vi "Inficon_Manual_HHV.vi"(5 "HHV-NG-Manual":sgl=1069.0, 6 "Manual HHV":bool, 7 "HHV-LP-Manual":sgl=2548.0, 8 "error in (no error)":errorcluster, 10 "Inficon_LP":refnum<queue>, 11 "Inficon_NG":refnum<queue>) -> (0 "error out":errorcluster)   [LabVIEW 2023]
uses:
  Tenney/support/Message Queue/Message Cluster.ctl
  Tenney/support/Message Queue/Enqueue Message (Single).vi
  Tenney/support/Message Queue/Tenney Message Queue.lvlib
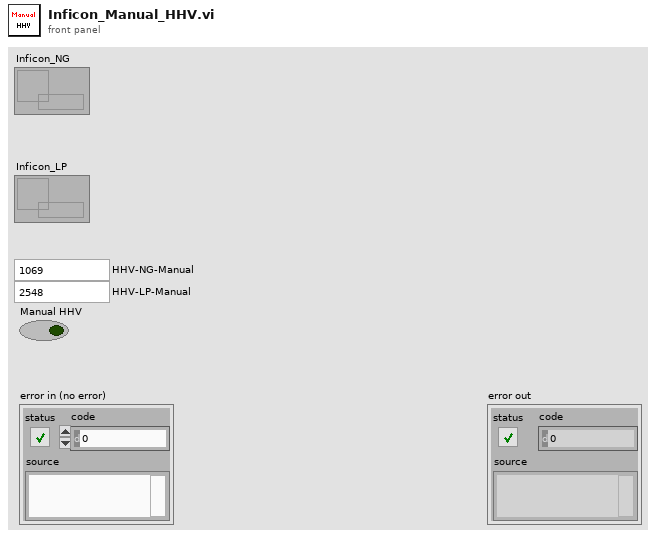
[diagram p1: front panel]
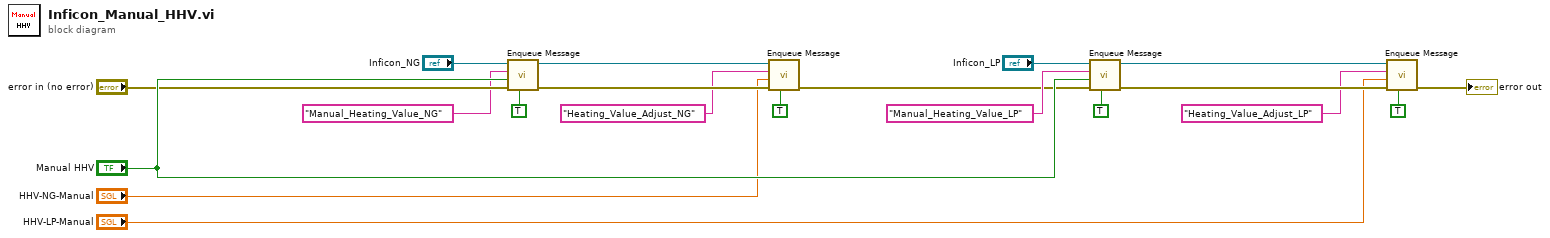
[diagram p0: block diagram]
diagram:
  n1 = call-poly "Enqueue Message.vi"("Priority Message? (F)"=TRUE, "error in (no error)"="error in (no error)", "Message Data"="Manual HHV", "Message"="Manual_Heating_Value_NG", "Message Queue"="Inficon_NG") -> ("error out"=w11:errorcluster, "dup Message Queue"=w9:refnum<queue>)  [unwired: 5 in]
  n2 = call-poly "Enqueue Message.vi"("Priority Message? (F)"=TRUE, "error in (no error)"=w11, "Message Data"="HHV-NG-Manual", "Message"="Heating_Value_Adjust_NG", "Message Queue"=w9) -> ("error out"=w10:errorcluster)  [unwired: 5 in, 1 out]
  n3 = call-poly "Enqueue Message.vi"("Priority Message? (F)"=TRUE, "error in (no error)"=w10, "Message Data"="Manual HHV", "Message"="Manual_Heating_Value_LP", "Message Queue"="Inficon_LP") -> ("error out"=w6:errorcluster, "dup Message Queue"=w5:refnum<queue>)  [unwired: 5 in]
  n4 = call-poly "Enqueue Message.vi"("Priority Message? (F)"=TRUE, "error in (no error)"=w6, "Message Data"="HHV-LP-Manual", "Message"="Heating_Value_Adjust_LP", "Message Queue"=w5) -> ("error out"=→"error out":errorcluster)  [unwired: 5 in, 1 out]
